vi "URAPI_WriteDigitalOut_num.vi"(0 "Value":enum16{"LO", "HI"}(ring)=enum."HI", 3 "URAPI Script":T1={"Script"="", "Whiles"=[], "Ifs"=[], "Supress Err"=TRUE, "Errors"=""}, 4 "Channel":u8) -> (2 "Variable Out":string, 5 "URAPI Script":T1={"Script"="", "Whiles"=[], "Ifs"=[], "Supress Err"=TRUE, "Errors"=""})   [LabVIEW 2014]
doc: "Writes the value of \"Variable In\" to the specified digital \"Channel\"."
uses:
  <userlib>/botspeak/VIs/Direct/URAPI_Control.ctl
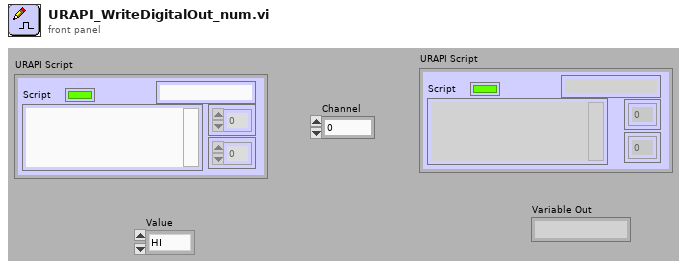
[diagram p1: front panel]
types:
  T1 = typedef "URAPI_Control.ctl" = cluster{"Script":string, "Whiles":u8[], "Ifs":u8[], "Supress Err":bool, "Errors":string}
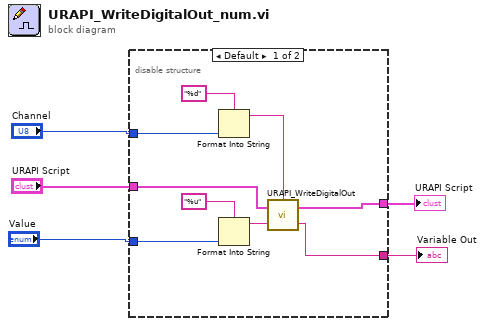
[diagram p0: block diagram]
diagram:
  n1 = disable-structure shown="Default" {
    disable-tunnel: "Channel" -> [w14 _]
    disable-tunnel: "URAPI Script" -> [w13 _]
    disable-tunnel: [w12 _] -> w3
    disable-tunnel: "Value" -> [w9 _]
    disable-tunnel: [w7 _] -> w1
    frame condition #0 (active) {
      n2 = Format Into String(format string="%d", w14) -> (resulting string=w11:string)  [unwired: 2 in, 1 out]
      n3 = Format Into String(format string="%u", w9) -> (resulting string=w6:string)  [unwired: 2 in, 1 out]
      n4 = call <userlib>:"URAPI_WriteDigitalOut.vi"("Variable In"=w6, "URAPI Script"=w13, "Channel"=w11) -> ("Variable Out"=w7:string, "URAPI Script"=w12:T1)  [unwired: 1 in]
    }
    frame condition #1 {
    }
  }
  "URAPI Script" <- w3
  "Variable Out" <- w1
